vi "GestioneFernoSubVI1.vi"(6 "ARRAY IMPOSTAZIONI INV.FRENI":T2[](array[typedef]) {"Controllo RPM"."Precisione pid Rpm" format="%#_13g"; "Controllo RPM"."PID gains Rpm"."derivative time (Td, min)" format="%.3f"; "Controllo RPM"."PID gains Rpm"."integral time (Ti, min)" format="%.3f"; "Controllo RPM"."PID gains Rpm"."proportional gain (Kc)" format="%.3f"; "Controllo potenza"."Precisione pid W" format="%#_13g"; "Controllo potenza"."PID gains potenza"."derivative time (Td, min)" format="%.3f"; "Controllo potenza"."PID gains potenza"."integral time (Ti, min)" format="%.3f"; "Controllo potenza"."PID gains potenza"."proportional gain (Kc)" format="%.3f"; "Controllo coppia"."Precisione pid Nm" format="%#_13g"; "Controllo coppia"."PID gains Coppia"."derivative time (Td, min)" format="%.3f"; "Controllo coppia"."PID gains Coppia"."integral time (Ti, min)" format="%.3f"; "Controllo coppia"."PID gains Coppia"."proportional gain (Kc)" format="%.3f"; "Compensa coppia residua"."PID gains C-RPM"."derivative time (Td, min)" format="%.3f"; "Compensa coppia residua"."PID gains C-RPM"."integral time (Ti, min)" format="%.3f"; "Compensa coppia residua"."PID gains C-RPM"."proportional gain (Kc)" format="%.3f"}, 7 "Array stato freni":T1[](array[typedef]) {"Rif AO coppia freno[Nm]" format="%#_13g"}, 9 "C max":dbl, 10 "Comandi freno":T1[](array[typedef]) {"Rif AO coppia freno[Nm]" format="%#_13g"}, 11 "Forza rif":bool) -> ()   [LabVIEW 2019]
uses:
  TypeDef/Stato_inverter.ctl
  TypeDef/InverterFreno.ctl
  cDAQ_PLC Folder/cDAQ/SET SINGLE AO.ctl
  cDAQ_PLC Folder/cDAQ/AO List.ctl
  cDAQ_PLC Folder/cDAQ/SET SINGLE DO.ctl
  cDAQ_PLC Folder/cDAQ/DO List.ctl
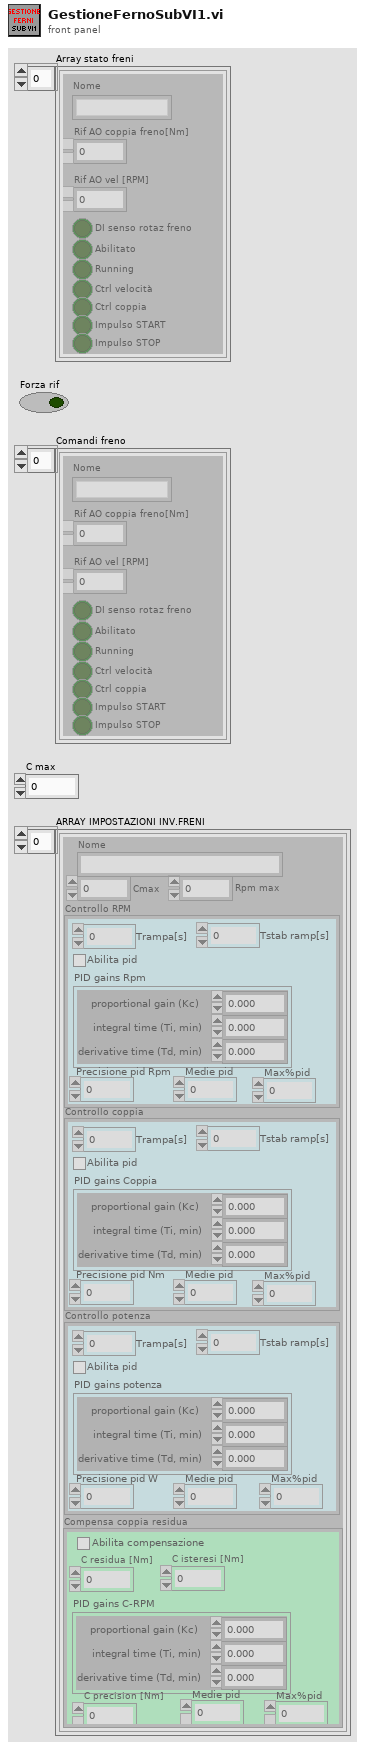
[diagram p1: front panel]
types:
  T1 = typedef "Stato_inverter.ctl" = cluster{"DI senso rotaz freno":bool, "Rif AO vel [RPM]":dbl, "Rif AO coppia freno[Nm]":dbl, "Abilitato":bool, "Running":bool, "Ctrl velocità":bool, "Nome":string, "Ctrl coppia":bool, "Impulso START":bool, "Impulso STOP":bool}
  T2 = typedef "InverterFreno.ctl" = cluster{"Nome":string, "Cmax":dbl, "Rpm max":dbl, "Compensa coppia residua":cluster{"Abilita compensazione":bool, "C residua [Nm]":dbl, "C isteresi [Nm]":dbl, "PID gains C-RPM":cluster{"proportional gain (Kc)":dbl, "integral time (Ti, min)":dbl, "derivative time (Td, min)":dbl}, "C precision [Nm]":dbl, "Max%pid":i32, "Medie pid":i32}, "Controllo coppia":cluster{"PID gains Coppia":cluster{"proportional gain (Kc)":dbl, "integral time (Ti, min)":dbl, "derivative time (Td, min)":dbl}, "Abilita pid":bool, "Precisione pid Nm":dbl, "Medie pid":i32, "Trampa[s]":i32, "Tstab ramp[s]":i32, "Max%pid":i32}, "Controllo potenza":cluster{"PID gains potenza":cluster{"proportional gain (Kc)":dbl, "integral time (Ti, min)":dbl, "derivative time (Td, min)":dbl}, "Abilita pid":bool, "Precisione pid W":dbl, "Medie pid":i32, "Trampa[s]":i32, "Tstab ramp[s]":i32, "Max%pid":i32}, "Controllo RPM":cluster{"PID gains Rpm":cluster{"proportional gain (Kc)":dbl, "integral time (Ti, min)":dbl, "derivative time (Td, min)":dbl}, "Abilita pid":bool, "Precisione pid Rpm":dbl, "Medie pid":i32, "Trampa[s]":i32, "Tstab ramp[s]":i32, "Max%pid":i32}}
  T3 = typedef "SET SINGLE DO.ctl" = cluster{"DO":T4, "Value":bool}
  T4 = typedef "DO List.ctl" = enum16{"OFF: ALL DO", "*ABILITA freno 1", "*ABILITA freno 2", "*ABILITA freno 3", "*START freno 1", "*START freno 2", "*START freno 3", "*STOP freno 1", "*STOP freno 3", "*STOP freno 2", "*Senso rot freno 1", "*Senso rot freno 2", "*Senso rot freno 3", "*Ctrl velocità freno 1", "*Ctrl velocità freno 2", "*Ctrl velocità freno 3", "*Ctrl coppia freno 1", "*Ctrl coppia freno 2", "*Ctrl coppia freno 3", "*ABILITA alimentatore 1", "*ABILITA alimentatore 2", "*ABILITA alimentatore 3", "*ABILITA alimentatore 4", "*START alimentatore 1", "*START alimentatore 2", "*START alimentatore 3", "*START alimentatore 4", "*STOP alimentatore 1", "*STOP alimentatore 2", "*STOP alimentatore 3", "*STOP alimentatore 4", "SENSO ROT alimentatore 1", "SENSO ROT alimentatore 2", "Abilita LEM 1000A", "Abilita LEM 300A", "Abilita sensori EXT WT", "B1 Seleziona linea 1", "B1 Seleziona linea 2", "B1 Seleziona linea 3", "B1 Seleziona linea 4", "B1 Seleziona linea 5", "B2 Seleziona linea 1", "B2 Seleziona linea 2", "B2 Seleziona linea 3", "B2 Seleziona linea 4", "B2 Seleziona linea 5", "*Reset allarmi", "*Start potenza AC", "*Stop potenza AC", "*Start potenza DC", "*Stop potenza DC", "*Start potenza DC eccit", "*Stop pontenza DC eccit", "Bypass res meter", "2nd canale res meter", "Enable res meter", "*Abilit teler ramo WT", "*Abil teler ramo princ Resit", "*Abil teler ramo 1 Resist", "*Abil teler ramo 2 Resist", "*Abil teler ramo 3 Resist", "*Abil cortocirc avvolgim", "*Controllo torsiometro B1", "*Controllo Torsiom B2", "*Scala torsiometro B1", "*Scala torsiometro B2", "*Collaudo in corso", "*Allarme presente", "Abilitazione elettroserratura", "Exit", "*Abilita collaudo", "*Abilita potenza trifase", "*Abilita potenza monofase", "*Abilita potenza DC", "*Abilita potenza DC eccit", "*Disabilita teleruttori potenza", "Set teleruttori prova a freddo", "Prova a freddo monofase", "Watchdog", "Forza DO PLC 3", "Forza DO PLC 2", "Forza DO PLC 1", "Forza DO cDAQ", "Scala 2000(T) 200(F) res meter", "Seleziona banco 1", "Seleziona banco 2", "Comando azionam in blocco", "Comando azionam reset", "Sensibilità freno 16 32 nm", "Reset Allarmi", "Carico res - Ramo 1", "Carico res - Ramo 2", "Carico res - Ramo 3", "Carico res - Ramo 4", "Carico res - Ramo 5", "Carico res - Ramo 6", "Carico res - Ramo 7", "Carico res - Ramo 8", "Carico res - Ramo 9", "Carico res - Ramo 10", "Carico res - Ramo 11", "Carico res - Start ventilatore", "Carico res - Stop ventilatore", "Abilita potenza solo freno", "Abilita AFE + freno trasc", "Abilita potenza carico resistivo", "Chiudi potenza AFE", "Apri potenza AFE", "Start AFE", "Config Banco2 TDE", "Misura diretto WT", "Ripristina centralina protezioni", "Abilita Scrittura Dati Keb", "Bench Selection(0-B1,1-B2)", "Select current mode", "Select toruqe mode", "Select speed mode", "Extenal alarm", "Enable Extenal program ", "Start ", "Stop", "Enable force mode", "Abilita linea 125 A", "Abilita linea 63 A", "Abilita linea 16 A", "Aum Tensione Variac", "Dim Tesnione Variac", "Abilita Ellecto Stractura", "Riprinto Emergenxe ", "Abilita Collaudo", "Disabilita Collaudo", "Abilita Ingresso Variac", "Abilita Uscita Variac", "Abilita ventilatore Variac"}
  T5 = typedef "SET SINGLE AO.ctl" = cluster{"AO":T6, "Value":dbl}
  T6 = typedef "AO List.ctl" = enum16{"OFF: ALL AO", "RIF VEL FRENO 1", "RIF VEL FRENO 2", "RIF VEL FRENO 3", "RIF COPPIA FRENO 1", "RIF COPPIA FRENO 2", "RIF COPPIA FRENO 3", "RIF V ALIM 1", "RIF F ALIM 1", "RIF V ALIM 2", "RIF F ALIM 2", "RIF V ALIM 3", "RIF F ALIM 3", "RIF V ALIM 4", "RIF F ALIM 4", "FORZA AO PLC 3", "FORZA AO PLC 2", "FORZA AO PLC 1", "FORZA AO cDAQ", "Configura alimentatore keb", "Tempo rampa keb", "Condensatori", "Exit"}
  T7 = cluster{"DI senso rotaz freno":bool, "Rif AO vel [RPM]":bool, "Rif AO coppia freno[Nm]":bool, "Abilitato":bool, "Running":bool, "Ctrl velocità":bool, "Nome":bool, "Ctrl coppia":bool, "Impulso START":bool, "Impulso STOP":bool}
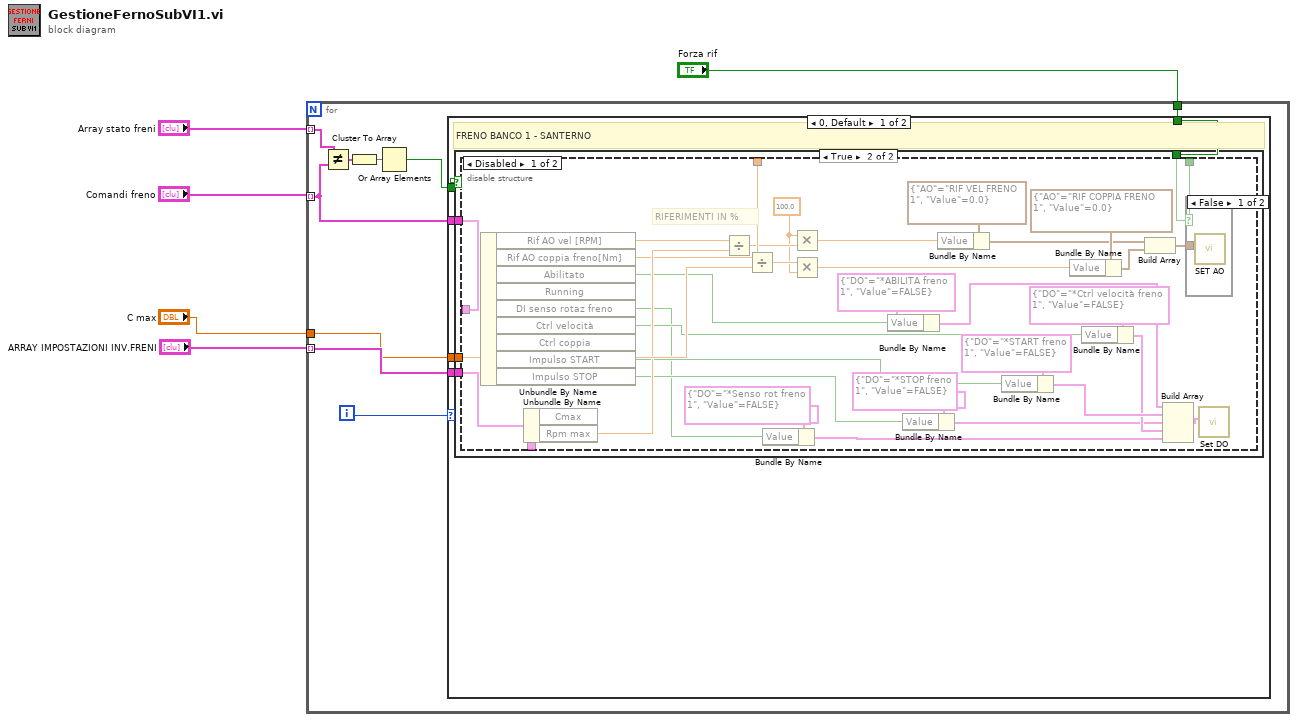
[diagram p0: block diagram]
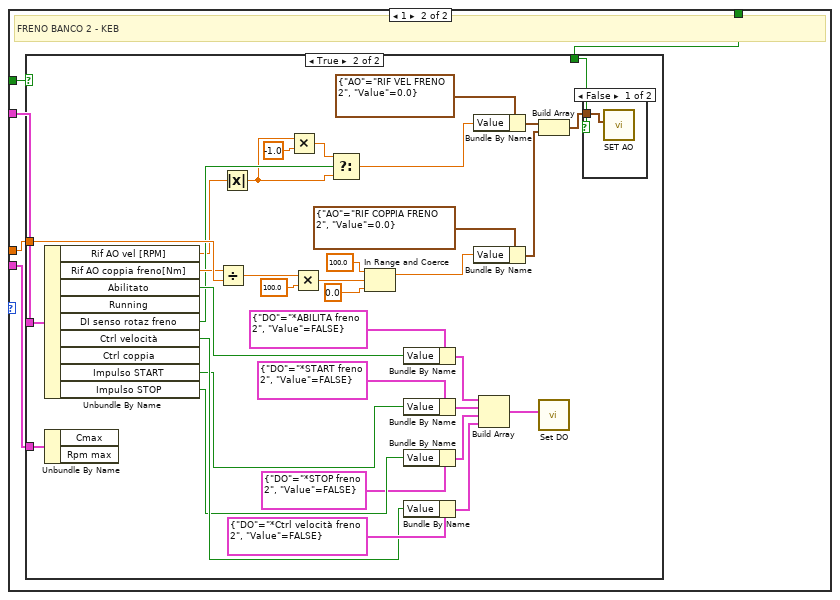
[diagram p5: hidden frame]
diagram:
  n1 = for {
    tunnel: "Comandi freno" -> [w13] mode=indexing
    tunnel: "Array stato freni" -> [w12] mode=indexing
    tunnel: "ARRAY IMPOSTAZIONI INV.FRENI" -> [w9] mode=indexing
    tunnel: "C max" -> [w8]
    tunnel: "Forza rif" -> [w6]
    i -> [w10]
    n2 = Not Equal?(x=w12, y=w13) -> (x != y?=w14:T7)
    n3 = Cluster To Array(cluster=w14) -> (array=w11:bool[])
    n4 = Or Array Elements(Boolean array=w11) -> (logical OR=w7:bool)
    n5 = case shown="0, Default" w10 {
      tunnel: w13 -> [w19 w62]
      tunnel: w7 -> [w18 w61]
      tunnel: w9 -> [w17 w60]
      tunnel: w8 -> [w16 w59]
      tunnel: w6 -> [w15 w58]
      frame 0, Default {
        # "FRENO BANCO 1 - SANTERNO"
        n6 = case shown="True" w18 {
          tunnel: w19 -> [_ w23]
          tunnel: w17 -> [_ w22]
          tunnel: w16 -> [_ w21]
          tunnel: w15 -> [_ w20]
          frame False {
          }
          frame True {
            n7 = disable-structure shown="Disabled" {
              disable-tunnel: w23 -> [w56 _]
              disable-tunnel: w22 -> [w46 _]
              disable-tunnel: w21 -> [w37 _]
              disable-tunnel: w20 -> [w24 _]
              frame Disabled {
                w41 = 100.0 ("x")
                # "RIFERIMENTI IN %"
                n8 = Unbundle By Name(w56) -> ("Rif AO vel [RPM]"=w45:dbl, "Rif AO coppia freno[Nm]"=w26:dbl, "Abilitato"=w36:bool, "DI senso rotaz freno"=w27:bool, "Ctrl velocità"=w38:bool, "Impulso START"=w33:bool, "Impulso STOP"=w29:bool)  [unwired: 2 out]
                n9 = Unbundle By Name(w46) -> ("Rpm max"=w43:dbl)  [unwired: 1 out]
                n10 = Divide(x=w45, y=w43) -> (x/y=w44:dbl)
                n11 = Divide(x=w26, y=w37) -> (x/y=w42:dbl)
                n12 = Bundle By Name(cluster=T3 {"DO"=enum."*Senso rot freno 1", "Value"=FALSE} ("Cluster SET DO"), "Value"=w27) -> (w39:T3)
                n13 = Multiply(x=w41, y=w44) -> (x*y=w25:dbl)
                n14 = Multiply(x=w42, y=w41) -> (x*y=w34:dbl)
                n15 = Bundle By Name(cluster=T3 {"DO"=enum."*ABILITA freno 1", "Value"=FALSE} ("Cluster SET DO"), "Value"=w36) -> (w32:T3)
                n16 = Bundle By Name(cluster=T3 {"DO"=enum."*STOP freno 1", "Value"=FALSE} ("Cluster SET DO"), "Value"=w29) -> (w30:T3)
                n17 = Bundle By Name(cluster=T5 {"AO"=enum."RIF VEL FRENO 1", "Value"=0.0} ("Cluster SET AO"), "Value"=w25) -> (w52:T5)
                n18 = Bundle By Name(cluster=T3 {"DO"=enum."*START freno 1", "Value"=FALSE} ("Cluster SET DO"), "Value"=w33) -> (w48:T3)
                n19 = Bundle By Name(cluster=T5 {"AO"=enum."RIF COPPIA FRENO 1", "Value"=0.0} ("Cluster SET AO"), "Value"=w34) -> (w51:T5)
                n20 = Bundle By Name(cluster=T3 {"DO"=enum."*Ctrl velocità freno 1", "Value"=FALSE} ("Cluster SET DO"), "Value"=w38) -> (w31:T3)
                n21 = Build Array(w52, w51) -> (w55:T5[])
                n22 = Build Array(w32, w48, w30, w31, w39) -> (w47:T3[])
                n23 = case shown="False" w24 {
                  tunnel: w55 -> [w57 _]
                  frame False {
                    n24 = call "SET AO.vi"("Cluster SET AO"=w57) -> ()  [unwired: 10 in, 1 out]
                  }
                  frame True {
                  }
                }
                n25 = call "Set DO.vi"("Cluster SET DO"=w47) -> ()  [unwired: 10 in, 1 out]
              }
              frame Enabled {
              }
            }
          }
        }
      }
      frame 1 {
        # "FRENO BANCO 2 - KEB"
        n26 = case shown="True" w61 {
          tunnel: w62 -> [_ w97]
          tunnel: w60 -> [_ w87]
          tunnel: w59 -> [_ w83]
          tunnel: w58 -> [_ w64]
          frame False {
          }
          frame True {
            n27 = Unbundle By Name(w97) -> ("Rif AO vel [RPM]"=w66:dbl, "Rif AO coppia freno[Nm]"=w74:dbl, "Abilitato"=w82:bool, "DI senso rotaz freno"=w69:bool, "Ctrl velocità"=w84:bool, "Impulso START"=w80:bool, "Impulso STOP"=w76:bool)  [unwired: 2 out]
            n28 = Unbundle By Name(w87) -> ()  [unwired: 2 out]
            n29 = Divide(x=w74, y=w83) -> (x/y=w86:dbl)
            n30 = Absolute Value(x=w66) -> (abs(x)=w63:dbl)
            n31 = Multiply(x=w63, y=-1.0) -> (x*y=w67:dbl)
            n32 = Multiply(x=w86, y=100.0 ("x")) -> (x*y=w73:dbl)
            n33 = Select(t=w67, s=w69, f=w63) -> (s? t:f=w68:dbl)
            n34 = In Range and Coerce(upper limit=100.0 ("lower limit"), x=w73, lower limit=0.0) -> (coerced(x)=w72:dbl)  [unwired: 1 out]
            n35 = Bundle By Name(cluster=T3 {"DO"=enum."*ABILITA freno 2", "Value"=FALSE} ("Cluster SET DO"), "Value"=w82) -> (w79:T3)
            n36 = Bundle By Name(cluster=T3 {"DO"=enum."*START freno 2", "Value"=FALSE} ("Cluster SET DO"), "Value"=w80) -> (w89:T3)
            n37 = Bundle By Name(cluster=T3 {"DO"=enum."*STOP freno 2", "Value"=FALSE} ("Cluster SET DO"), "Value"=w76) -> (w77:T3)
            n38 = Bundle By Name(cluster=T3 {"DO"=enum."*Ctrl velocità freno 2", "Value"=FALSE} ("Cluster SET DO"), "Value"=w84) -> (w78:T3)
            n39 = Bundle By Name(cluster=T5 {"AO"=enum."RIF VEL FRENO 2", "Value"=0.0} ("Cluster SET AO"), "Value"=w68) -> (w93:T5)
            n40 = Bundle By Name(cluster=T5 {"AO"=enum."RIF COPPIA FRENO 2", "Value"=0.0} ("Cluster SET AO"), "Value"=w72) -> (w92:T5)
            n41 = Build Array(w79, w89, w77, w78) -> (w88:T3[])
            n42 = Build Array(w93, w92) -> (w96:T5[])
            n43 = call "Set DO.vi"("Cluster SET DO"=w88) -> ()  [unwired: 10 in, 1 out]
            n44 = case shown="False" w64 {
              tunnel: w96 -> [w98 _]
              frame False {
                n45 = call "SET AO.vi"("Cluster SET AO"=w98) -> ()  [unwired: 10 in, 1 out]
              }
              frame True {
              }
            }
          }
        }
      }
    }
  }
